vi "OrderExecuted.vi"(11 "buffer.in":u64[](array[numeric])=[0, 0, 0, 0, 0, 0, 0, 0, 0] format="%.0x") -> (3 "OrderBook.Command":T1)   [LabVIEW 2022 SP3]
uses:
  common/orderbook.command.ctl
  common/orderbook.command.type.ctl
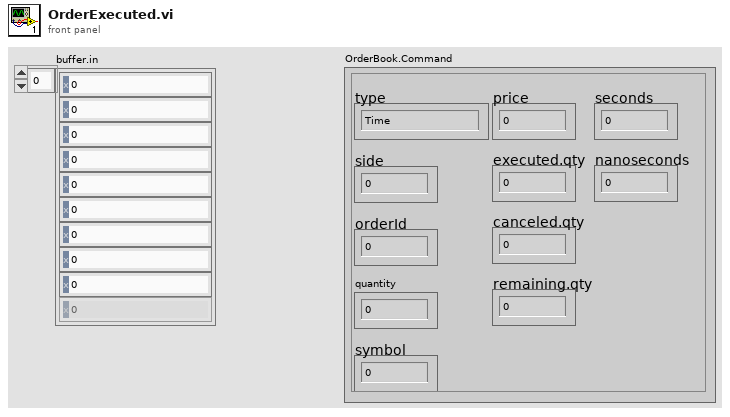
[diagram p1: front panel]
types:
  T1 = typedef "orderbook.command.ctl" = cluster{"type":T2, "side":u8, "orderId ":u64, "quantity":u32, "symbol":u64, "price":u64, "executed.qty":u32, "canceled.qty":u32, "remaining.qty":u32, "seconds":u64, "nanoseconds":u64}
  T2 = typedef "orderbook.command.type.ctl" = enum8{"Time", "AddOrder", "OrderExecuted", "OrderExecutedAtPrice", "ReduceSize", "ModifyOrder", "DeleteOrder", "Get.State", "Get.All.Orders", "Get.Top"}
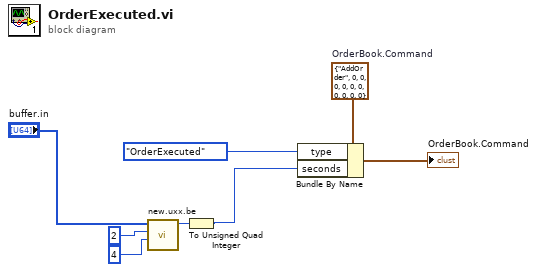
[diagram p0: block diagram]
diagram:
  w3 = T1 {"type"=enum."AddOrder", "side"=0, "orderId "=0, "quantity"=0, "symbol"=0, "price"=0, "executed.qty"=0, "canceled.qty"=0, "remaining.qty"=0, "seconds"=0, "nanoseconds"=0}  # OrderBook.Command
  n1 = call "new.uxx.be.vi"("buffer (U64)"="buffer.in", "Start.Idx"=u8 2, "Length"=u8 4) -> ("Uxx.be"=w4:u64)  [unwired: 7 in]
  n2 = To Unsigned Quad Integer(1:w4) -> (0:w8:u64)
  n3 = Bundle By Name(cluster=w3, "type"=orderbook.command.type."OrderExecuted" ("OrderBook Command"), "seconds"=w8) -> (→"OrderBook.Command":T1)
